vi "WriteFile.vi"(6 "Overwrite?(F)":bool, 8 "error in (no error)":errorcluster, 9 "Proposed File Name":string, 10 "Output Path":path, 11 "CarexData In":refnum<class "ExpData.lvclass">) -> (0 "error out":errorcluster, 1 "Actual File Name":string, 3 "CarexData Out":refnum<class "ExpData.lvclass">)   [LabVIEW 2015, in "ExpData.lvclass"]
uses:
  ExpData.lvclass
  ExpData.lvclass/ExpData.ctl
  <vilib>/Utility/file.llb/Write To Spreadsheet File (DBL).vi
  CustomVIs/CustomVI.lvlib
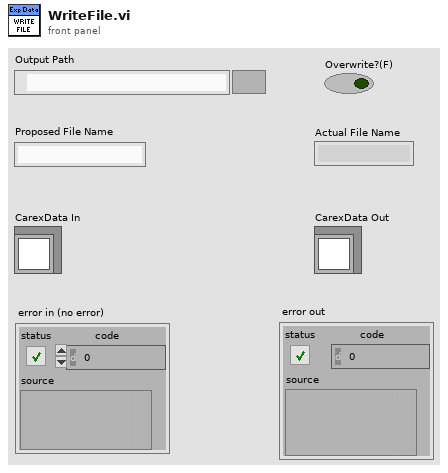
[diagram p1: front panel]
types:
  T1 = enum16{"Native", "Native Command Line", "UNIX", "Macintosh", "DOS"}
  T2 = enum16{"open", "replace", "create", "open or create", "replace or create", "replace or create with confirmation"}
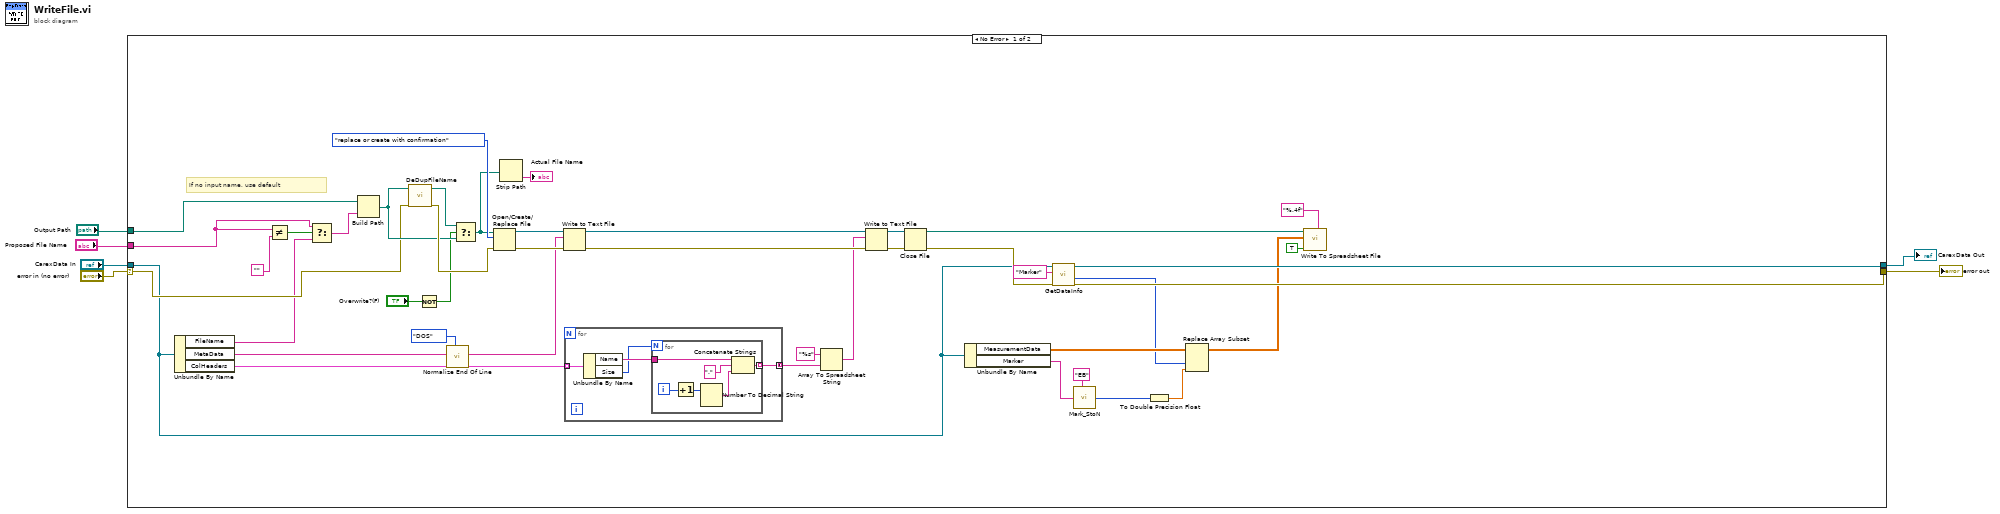
[diagram p0: block diagram]
diagram:
  n1 = case shown="No Error" "error in (no error)" {
    selector: "error in (no error)" -> [w34 w61]
    tunnel: [w23 w60] -> w5
    tunnel: [w21 w61] -> w6
    tunnel: "Output Path" -> [w43 _]
    tunnel: "CarexData In" -> [w13 w60]
    tunnel: "Proposed File Name" -> [w47 _]
    frame No Error {
      # "If no input name, use default"
      n2 = Unbundle By Name(w13) -> ("FileName"=w12:string, "MetaData"=w10:string, "ColHeaders"=w11:cluster{"Name":string, "Index":i8, "Size":i8}[])
      n3 = Not Equal?(x=w47, y="") -> (x != y?=w48:bool)
      n4 = Select(t=w47, s=w48, f=w12) -> (s? t:f=w42:string)
      n5 = Build Path(base path=w43, name or relative path=w42) -> (appended path=w40:path)
      n6 = call "DeDupFileName.vi"("error in (no error)"=w34, "Path"=w40) -> ("error out"=w41:errorcluster, "Out Path"=w46:path)  [unwired: 7 in, 1 out]
      n7 = Not(x="Overwrite?(F)") -> (.not. x?=w39:bool)
      n8 = call <vilib>:"Normalize End Of Line.vi"("end of line (Native)"=T1."DOS", "string in"=w10) -> ("string out"=w9:string)  [unwired: 6 in]
      n9 = Select(t=w46, s=w39, f=w40) -> (s? t:f=w37:path)
      n10 = Open/Create/Replace File(file path (use dialog)=w37, error in=w41, operation (0:open)=T2."replace or create with confirmation") -> (refnum out=w15:refnum<file>, error out=w14:errorcluster)  [unwired: 3 in, 1 out]
      n11 = Strip Path(path=w37) -> (name=→"Actual File Name":string)  [unwired: 1 out]
      n12 = Write to Text File(file (use dialog)=w15, text=w9, error in=w14) -> (refnum out=w33:refnum<file>, error out=w32:errorcluster)  [unwired: 1 in, 1 out]
      n13 = for {
        tunnel: w11 -> [w53] mode=indexing
        tunnel: [w50] -> w29 mode=concatenating
        n14 = Unbundle By Name(w53) -> ("Name"=w52:string, "Size"=w51:i8)
        n15 = for {
          N: w51 -> [_]
          tunnel: w52 -> [w56]
          tunnel: [w54] -> w50 mode=indexing
          i -> [w59]
          n16 = Increment(x=w59) -> (x+1=w58:i32)
          n17 = Number To Decimal String(number=w58) -> (decimal integer string=w57:string)  [unwired: 1 in]
          n18 = Concatenate Strings(w56, "." ("format string"), w57) -> (w54:string)
        }
      }
      n19 = Array To Spreadsheet String(array=w29, 3:"%s" ("format string")) -> (spreadsheet string=w27:string)  [unwired: 1 in]
      n20 = Write to Text File(file (use dialog)=w33, text=w27, error in=w32) -> (refnum out=w31:refnum<file>, error out=w30:errorcluster)  [unwired: 1 in, 1 out]
      n21 = Close File(refnum=w31, error in=w30) -> (path=w35:path, error out=w22:errorcluster)
      n22 = Unbundle By Name(w13) -> ("MeasurementData"=w19:dbl[][], "Marker"=w24:string[])
      n23 = call "GetDataInfo.vi"("error in (no error)"=w22, "Name"="Marker", "CarexMData in"=w13) -> ("error out"=w21:errorcluster, "Index"=w7:i8, "CarexMData out"=w23:refnum<class "ExpData.lvclass">)  [unwired: 4 in, 2 out]
      n24 = call "Mark_StoN.vi"("Marker(Low->High)"="EB", "MarkerString"=w24) -> ("MarkerNumber"=w18:u32[])  [unwired: 3 in]
      n25 = To Double Precision Float(number=w18) -> (double precision float=w17:dbl[])
      n26 = Replace Array Subset(array=w19, new element=w17, index (col)=w7) -> (w16:dbl[][])  [unwired: 1 in]
      n27 = call-poly <vilib>:"Write To Spreadsheet File.vi"("format (%.3f)"="%.4f", "append to file? (new file:F)"=TRUE, "2D data"=w16, "file path (dialog if empty)"=w35) -> ()  [unwired: 4 in, 1 out]
    }
    frame Error {
    }
  }
  "CarexData Out" <- w5
  "error out" <- w6
